vi "VelocityProfile.vi"(0 "t":dbl, 1 "a1":dbl=10.0, 3 "a3":dbl=15.0, 5 "s":dbl, 7 "intervalo":dbl=0.016, 9 "v_est":dbl, 11 "v_max":dbl=3.0, 12 "v3":dbl, 13 "s3":dbl) -> (4 "Velocity":dbl, 6 "VelocityProfileState Out":T1, 8 "Velocities":dbl[](array[numeric]), 10 "Time":dbl[](array[numeric]))   [LabVIEW 2018]
uses:
  Controle/VelocityProfileState.ctl
panel:
  in  "Amax":dbl=8.0
  in  "Reset":bool
  out "Velocity Profile":cluster{dbl[], dbl[]}(graph)
  in  "Tolerancia Vel":dbl=0.01
  in  "Tolerancia Pos":dbl=0.010000000000000004
  out "VelocityProfileState In":T1={"t0"=0.0, "t1"=0.0, "t2"=0.0, "t3"=0.0, "v0"=0.0, "v_max"=3.0, "v3"=0.0, "v2"=0.0, "v1"=0.0, "perfil"=enum."Triangular", "regiao"=0, "s0"=0.0, "s1"=0.0, "s2"=0.0, "v"=0.0, "t"=0.0, "a1"=10.0, "s3"=0.0, "Reset"=FALSE, "s"=0.0, "a3"=15.0, "Ré"=FALSE, "Impossível"=FALSE, "intervalo"=0.0}
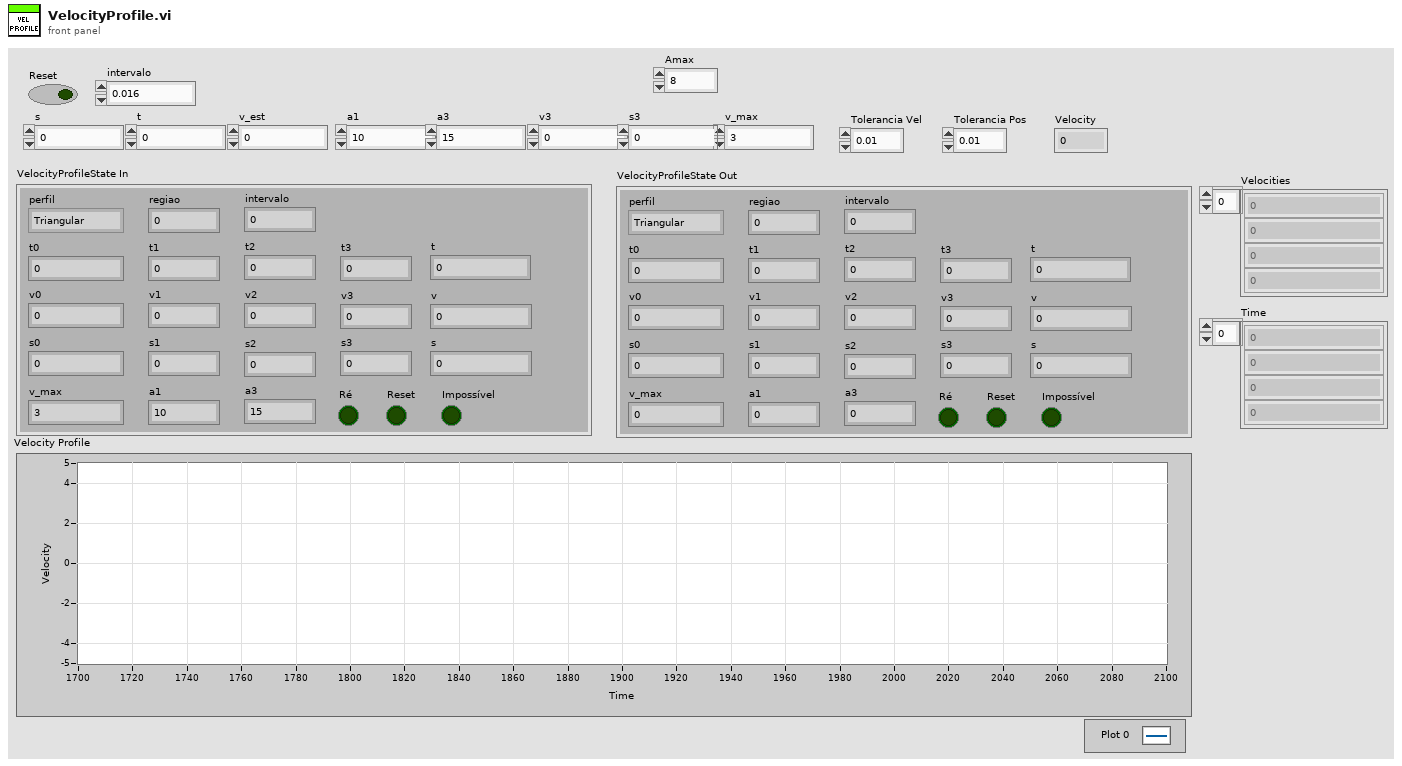
[diagram p1: front panel]
types:
  T1 = typedef "VelocityProfileState.ctl" = cluster{"t0":dbl, "t1":dbl, "t2":dbl, "t3":dbl, "v0":dbl, "v_max":dbl, "v3":dbl, "v2":dbl, "v1":dbl, "perfil":enum16{"Triangular", "Trapezoidal"}, "regiao":i32, "s0":dbl, "s1":dbl, "s2":dbl, "v":dbl, "t":dbl, "a1":dbl, "s3":dbl, "Reset":bool, "s":dbl, "a3":dbl, "Ré":bool, "Impossível":bool, "intervalo":dbl}
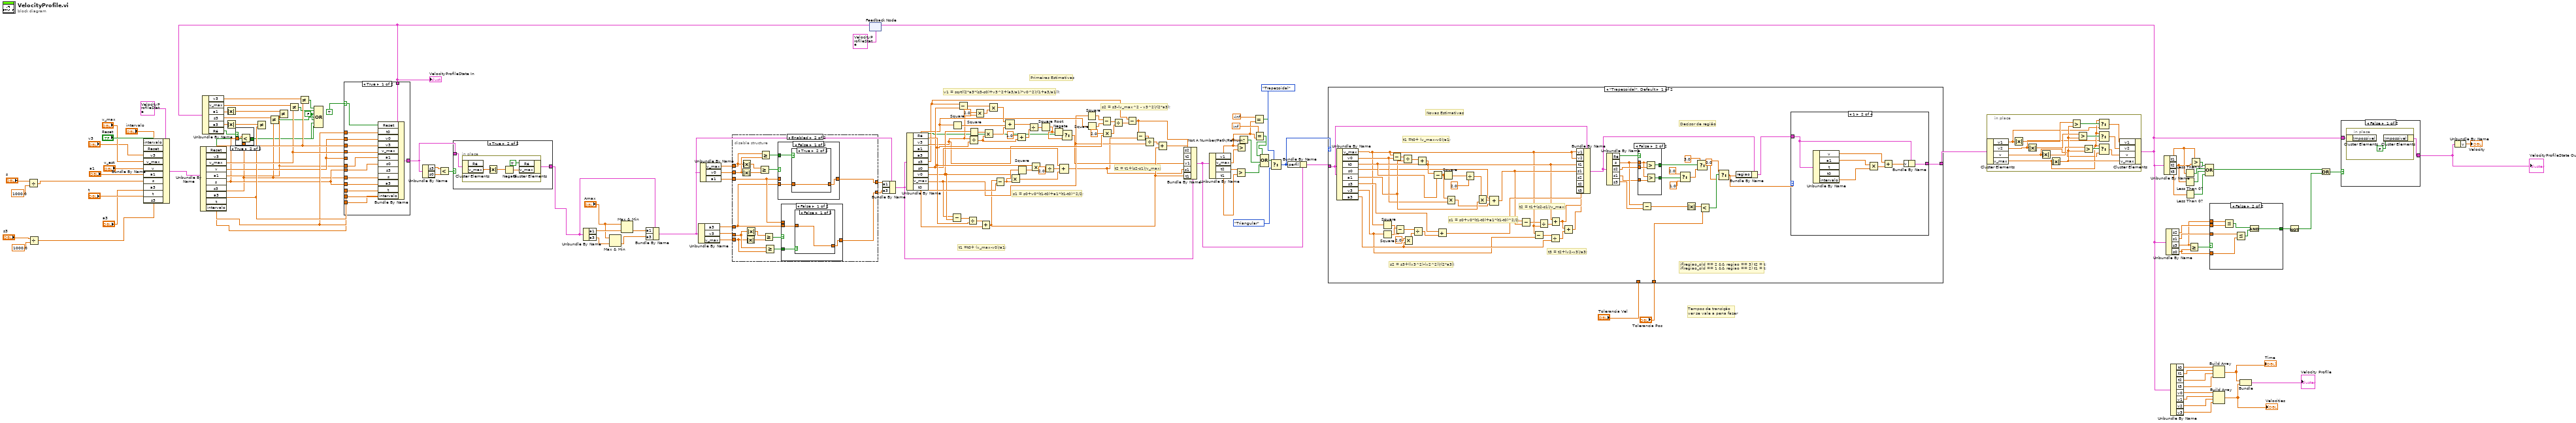
[diagram p0: block diagram]
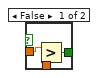
[diagram p2: hidden frame]
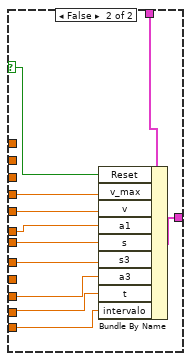
[diagram p3: hidden frame]
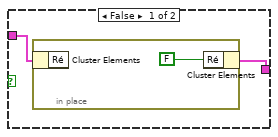
[diagram p4: hidden frame]
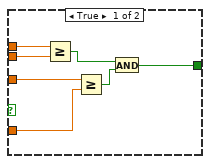
[diagram p5: hidden frame]
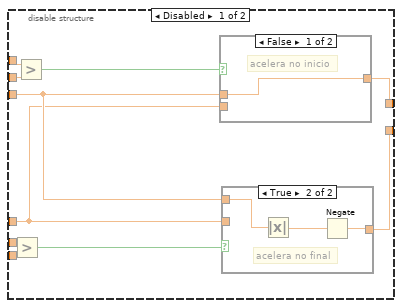
[diagram p6: hidden frame]
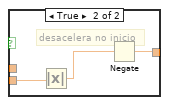
[diagram p8: hidden frame]
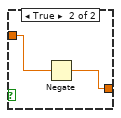
[diagram p9: hidden frame]
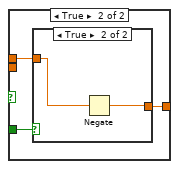
[diagram p10: hidden frame]
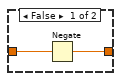
[diagram p12: hidden frame]
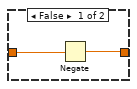
[diagram p14: hidden frame]
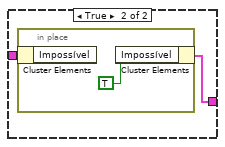
[diagram p15: hidden frame]
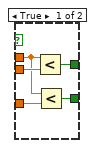
[diagram p16: hidden frame]
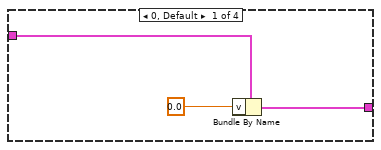
[diagram p17: hidden frame]
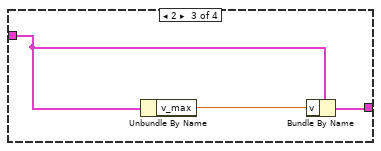
[diagram p18: hidden frame]
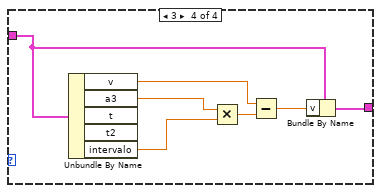
[diagram p19: hidden frame]
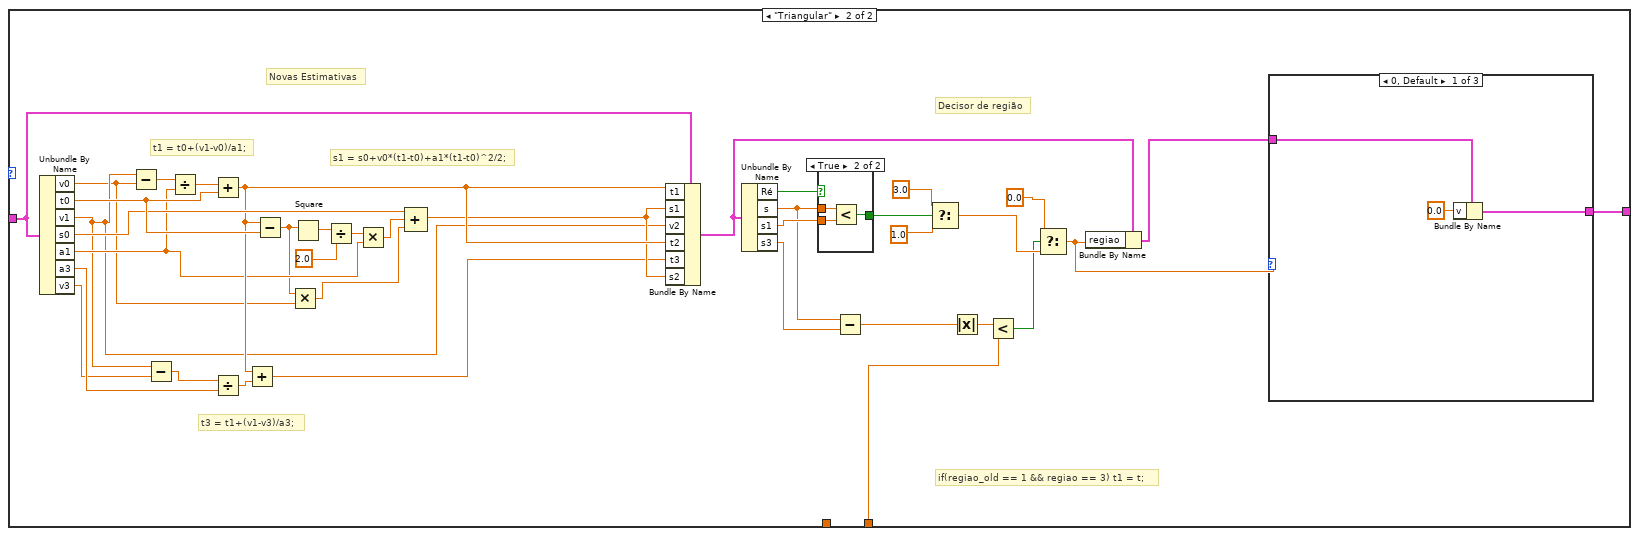
[diagram p20: hidden frame]
diagram:
  w37 = FALSE ("value")
  # "Tempos de transição\nver se vale a pena fazer"
  # "Primeiras Estimativas"
  # "t2 = t1+(s2-s1)/v_max;"
  # "s2 = s3-(v_max^2 - v3^2)/(2*a3);"
  # "s1 = s0+v0*(t1-t0)+a1*(t1-t0)^2/2;"
  # "t1 =t0+ (v_max-v0)/a1;"
  # "v1 = sqrt((2*a3*(s3-s0)+v3^2+(a3/a1)*v0^2)/(1+a3/a1));"
  n1 = Divide(x="s", y=1000.0) -> (x/y=w6:dbl)
  n2 = Divide(x="s3", y=1000.0) -> (x/y=w7:dbl)
  n3 = Bundle By Name(cluster=T1 {"t0"=0.0, "t1"=0.0, "t2"=0.0, "t3"=0.0, "v0"=0.0, "v_max"=0.0, "v3"=0.0, "v2"=0.0, "v1"=0.0, "perfil"=enum."Triangular", "regiao"=0, "s0"=0.0, "s1"=0.0, "s2"=0.0, "v"=0.0, "t"=0.0, "a1"=0.0, "s3"=0.0, "Reset"=FALSE, "s"=0.0, "a3"=0.0, "Ré"=FALSE, "Impossível"=FALSE, "intervalo"=0.0} ("VelocityProfileState In"), "intervalo"="intervalo", "Reset"="Reset", "v3"="v3", "v_max"="v_max", "v"="v_est", "a1"="a1", "s"=w6, "a3"="a3", "t"="t", "s3"=w7) -> (w43:T1)
  n4 = Unbundle By Name(w43) -> ("Reset"=w39:bool, "v3"=w135:dbl, "v_max"=w133:dbl, "v"=w63:dbl, "a1"=w62:dbl, "s"=w41:dbl, "s3"=w40:dbl, "a3"=w67:dbl, "t"=w64:dbl, "intervalo"=w31:dbl)
  n5 = feedback #1(T1 {"t0"=0.0, "t1"=0.0, "t2"=0.0, "t3"=0.0, "v0"=0.0, "v_max"=0.0, "v3"=0.0, "v2"=0.0, "v1"=0.0, "perfil"=enum."Triangular", "regiao"=0, "s0"=0.0, "s1"=0.0, "s2"=0.0, "v"=0.0, "t"=0.0, "a1"=0.0, "s3"=0.0, "Reset"=FALSE, "s"=0.0, "a3"=0.0, "Ré"=FALSE, "Impossível"=FALSE, "intervalo"=0.0} ("VelocityProfileState In")) -> (w19:T1)
  "VelocityProfileState In" <- w19
  n6 = Unbundle By Name(w19) -> ("v3"=w136:dbl, "v_max"=w134:dbl, "a1"=w46:dbl, "s3"=w132:dbl, "a3"=w45:dbl, "Ré"=w42:bool)
  n7 = Absolute Value(x=w46) -> (abs(x)=w47:dbl)
  n8 = Absolute Value(x=w45) -> (abs(x)=w44:dbl)
  n9 = case shown="True" w42 {
    tunnel: w41 -> [w158 w161]
    tunnel: w40 -> [w157 w160]
    tunnel: [w156 w159] -> w38
    frame False {
      n10 = Greater?(x=w158, y=w157) -> (0:w156:bool)
    }
    frame True {
      n11 = Less?(x=w161, y=w160) -> (x < y?=w159:bool)
    }
  }
  n12 = Not Equal?(x=w44, y=w67) -> ()  [unwired: 1 out]
  n13 = Not Equal?(x=w132, y=w40) -> (x != y?=w129:bool)
  n14 = Not Equal?(x=w47, y=w62) -> ()  [unwired: 1 out]
  n15 = Not Equal?(x=w134, y=w133) -> (x != y?=w130:bool)
  n16 = Not Equal?(x=w136, y=w135) -> (x != y?=w131:bool)
  n17 = Compound Arithmetic op=OR(w131, w130, w37, w129, w37, w38, w39) -> ()  [unwired: 1 out]
  n18 = case shown="True" TRUE {
    selector: TRUE -> [w169 w182]
    tunnel: w64 -> [w175 _]
    tunnel: w63 -> [w174 _]
    tunnel: w135 -> [w173 _]
    tunnel: w133 -> [w172 w186]
    tunnel: w63 -> [_ w185]
    tunnel: [w171 w184] -> w153
    tunnel: w19 -> [w170 w183]
    tunnel: w67 -> [w168 w181]
    tunnel: w64 -> [w167 w180]
    tunnel: w41 -> [w166 _]
    tunnel: w62 -> [w162 w179]
    tunnel: w41 -> [w165 w178]
    tunnel: w40 -> [w164 w177]
    tunnel: w31 -> [w163 w176]
    frame True {
      n19 = Bundle By Name(cluster=w170, "Reset"=w169, "t0"=w175, "v0"=w174, "v3"=w173, "v_max"=w172, "a1"=w162, "s0"=w165, "s3"=w164, "s"=w166, "a3"=w168, "t"=w167, "intervalo"=w163) -> (w171:T1)
    }
    frame False {
      n20 = Bundle By Name(cluster=w183, "Reset"=w182, "v_max"=w186, "v"=w185, "a1"=w179, "s"=w178, "s3"=w177, "a3"=w181, "t"=w180, "intervalo"=w176) -> (w184:T1)
    }
  }
  n21 = Unbundle By Name(w153) -> ("s3"=w155:dbl, "s0"=w154:dbl)
  n22 = Less?(x=w155, y=w154) -> (x < y?=w66:bool)
  n23 = case shown="True" w66 {
    tunnel: w153 -> [w188 w191]
    tunnel: [w187 w190] -> w15
    frame False {
      n24 = in-place {
        n25 = in-place-cluster #2(w188) -> ()  [unwired: 1 out]
        n26 = in-place-cluster #2("Ré"=FALSE) -> (w187:T1)
      }
    }
    frame True {
      n27 = in-place {
        n28 = in-place-cluster #3(w191) -> ("v_max"=w195:dbl)  [unwired: 1 out]
        n29 = Absolute Value(x=w195) -> (abs(x)=w194:dbl)
        n30 = Negate(x=w194) -> (-x=w193:dbl)
        n31 = in-place-cluster #3("Ré"=TRUE, "v_max"=w193) -> (w190:T1)
      }
    }
  }
  n32 = Unbundle By Name(w15) -> ("a1"=w14:dbl, "a3"=w11:dbl)
  n33 = Max & Min(x="Amax", y=w11) -> (min(x,y)=w10:dbl)  [unwired: 1 out]
  n34 = Max & Min(x="Amax", y=w14) -> (min(x,y)=w13:dbl)  [unwired: 1 out]
  n35 = Bundle By Name(cluster=w15, "a1"=w13, "a3"=w10) -> (w16:T1)
  n36 = Unbundle By Name(w16) -> ("a3"=w68:dbl, "v3"=w113:dbl, "v_max"=w114:dbl)
  n37 = Unbundle By Name(w16) -> ("v_max"=w152:dbl, "v0"=w151:dbl, "a1"=w69:dbl)
  n38 = disable-structure shown="Enabled" {
    disable-tunnel: w152 -> [w205 w225]
    disable-tunnel: w151 -> [w204 w224]
    disable-tunnel: w114 -> [w203 w216]
    disable-tunnel: w113 -> [w202 w217]
    disable-tunnel: [w200 w223] -> w71
    disable-tunnel: [w198 w218] -> w70
    disable-tunnel: w69 -> [w197 w215]
    disable-tunnel: w68 -> [w196 w214]
    frame Disabled {
      n39 = Greater?(x=w202, y=w203) -> (0:w199:bool)
      n40 = Greater?(x=w205, y=w204) -> (0:w201:bool)
      n41 = case shown="False" w201 {
        tunnel: [w210 w212] -> w200
        tunnel: w197 -> [w210 _]
        tunnel: w196 -> [_ w213]
        frame False {
          # "acelera no inicio"
        }
        frame True {
          # "desacelera no inicio"
          n42 = Absolute Value(x=w213) -> (abs(x)=w211:dbl)
          n43 = Negate(x=w211) -> (-x=w212:dbl)
        }
      }
      n44 = case shown="True" w199 {
        tunnel: [w206 w209] -> w198
        tunnel: w197 -> [_ w207]
        tunnel: w196 -> [w206 _]
        frame False {
          # "desacelera no final"
        }
        frame True {
          # "acelera no final"
          n45 = Absolute Value(x=w207) -> (abs(x)=w208:dbl)
          n46 = Negate(x=w208) -> (-x=w209:dbl)
        }
      }
    }
    frame Enabled {
      n47 = Absolute Value(x=w224) -> (abs(x)=w228:dbl)
      n48 = Absolute Value(x=w225) -> (abs(x)=w229:dbl)
      n49 = Absolute Value(x=w216) -> (abs(x)=w220:dbl)
      n50 = Absolute Value(x=w217) -> (abs(x)=w219:dbl)
      n51 = Greater Or Equal?(x=w229, y=w228) -> (x >= y?=w227:bool)
      n52 = Greater Or Equal?(x=w225, y=w224) -> (x >= y?=w226:bool)
      n53 = Greater Or Equal?(x=w219, y=w220) -> (x >= y?=w221:bool)
      n54 = Greater Or Equal?(x=w217, y=w216) -> (x >= y?=w222:bool)
      n55 = case shown="False" w227 {
        tunnel: w215 -> [_ w248]
        tunnel: w226 -> [w244 w250]
        tunnel: [w243 w249] -> w223
        tunnel: w214 -> [w242 _]
        frame False {
          n56 = case shown="True" w244 {
            tunnel: [w245 w247] -> w243
            tunnel: w242 -> [w246 w247]
            frame False {
              n57 = Negate(x=w246) -> (-x=w245:dbl)
            }
            frame True {
            }
          }
        }
        frame True {
          n58 = case shown="True" w250 {
            tunnel: [w251 w253] -> w249
            tunnel: w248 -> [w252 w253]
            frame False {
              n59 = Negate(x=w252) -> (-x=w251:dbl)
            }
            frame True {
            }
          }
        }
      }
      n60 = case shown="False" w221 {
        tunnel: w222 -> [w232 w238]
        tunnel: [w231 w237] -> w218
        tunnel: w215 -> [_ w236]
        tunnel: w214 -> [w230 _]
        frame False {
          n61 = case shown="False" w232 {
            tunnel: [w233 w234] -> w231
            tunnel: w230 -> [w233 w235]
            frame False {
            }
            frame True {
              n62 = Negate(x=w235) -> (-x=w234:dbl)
            }
          }
        }
        frame True {
          n63 = case shown="True" w238 {
            tunnel: [w239 w241] -> w237
            tunnel: w236 -> [w239 w240]
            frame False {
            }
            frame True {
              n64 = Negate(x=w240) -> (-x=w241:dbl)
            }
          }
        }
      }
    }
  }
  n65 = Bundle By Name(cluster=w16, "a1"=w71, "a3"=w70) -> (w72:T1)
  n66 = Unbundle By Name(w72) -> ("Ré"=w65:bool, "v3"=w87:dbl, "a1"=w105:dbl, "a3"=w84:dbl, "s3"=w81:dbl, "s0"=w104:dbl, "v0"=w103:dbl, "v_max"=w79:dbl, "t0"=w112:dbl)
  n67 = Subtract(x=w79, y=w103) -> (x-y=w150:dbl)
  n68 = Square(x=w87) -> (x^2=w100:dbl)
  n69 = Subtract(x=w81, y=w104) -> (x-y=w99:dbl)
  n70 = Divide(x=w150, y=w105) -> (x/y=w149:dbl)
  n71 = Divide(x=w84, y=w105) -> (x/y=w93:dbl)
  n72 = Square(x=w103) -> (x^2=w102:dbl)
  n73 = Multiply(x=2.0, y=w84) -> (x*y=w98:dbl)
  n74 = Add(x=w149, y=w112) -> (x+y=w77:dbl)
  n75 = Multiply(x=w102, y=w93) -> (x*y=w101:dbl)
  n76 = Multiply(x=w99, y=w98) -> (x*y=w96:dbl)
  n77 = Subtract(x=w77, y=w112) -> (x-y=w111:dbl)
  n78 = Compound Arithmetic op=ADD(w96, w100, w101) -> (w95:dbl)
  n79 = Multiply(x=w103, y=w111) -> (x*y=w106:dbl)
  n80 = Add(x=1.0, y=w93) -> (x+y=w94:dbl)
  n81 = Square(x=w111) -> (x^2=w110:dbl)
  n82 = Divide(x=w95, y=w94) -> (x/y=w91:dbl)
  n83 = Multiply(x=w105, y=w110) -> (x*y=w109:dbl)
  n84 = Square Root(x=w91) -> (sqrt(x)=w90:dbl)
  n85 = Divide(x=w109, y=2.0) -> (x/y=w107:dbl)
  n86 = Negate(x=w90) -> (-x=w117:dbl)
  n87 = Compound Arithmetic op=ADD(w104, w107, w106) -> (w73:dbl)
  n88 = Select(t=w117, s=w65, f=w90) -> (s? t:f=w74:dbl)
  n89 = Square(x=w79) -> (x^2=w89:dbl)
  n90 = Square(x=w87) -> (x^2=w88:dbl)
  n91 = Subtract(x=w89, y=w88) -> (x-y=w86:dbl)
  n92 = Multiply(x=2.0, y=w84) -> (x*y=w85:dbl)
  n93 = Divide(x=w86, y=w85) -> (x/y=w82:dbl)
  n94 = Subtract(x=w81, y=w82) -> (x-y=w76:dbl)
  n95 = Subtract(x=w76, y=w73) -> (x-y=w80:dbl)
  n96 = Divide(x=w80, y=w79) -> (x/y=w78:dbl)
  n97 = Add(x=w78, y=w77) -> (x+y=w75:dbl)
  n98 = Bundle By Name(cluster=w72, "s2"=w76, "t2"=w75, "v1"=w74, "s1"=w73, "t1"=w77) -> (w141:T1)
  n99 = Unbundle By Name(w141) -> ("v1"=w3:dbl, "v_max"=w148:dbl, "t2"=w147:dbl, "t1"=w146:dbl)
  n100 = Greater?(x=w147, y=w146) -> (0:w36:bool)
  n101 = Greater?(x=w3, y=w148) -> ()  [unwired: 1 out]
  n102 = Not A Number/Path/Refnum?(number/path/refnum=w3) -> (NaN/Path/Refnum?=w115:bool)
  n103 = Equal?(x=-inf, y=w3) -> (x = y?=w1:bool)
  n104 = Equal?(x=inf, y=w3) -> (x = y?=w35:bool)
  n105 = Compound Arithmetic op=OR(w1, w35, w115, w36) -> (w116:bool)
  n106 = Select(t=enum16{"Triangular", "Trapezoidal"}."Trapezoidal" ("perfil"), s=w116, f=enum16{"Triangular", "Trapezoidal"}."Triangular" ("perfil")) -> (s? t:f=w143:enum16{"Triangular", "Trapezoidal"})
  n107 = Bundle By Name(cluster=w141, "perfil"=w143) -> (w142:T1)
  n108 = case shown="\"Trapezoidal\", Default" w143 {
    tunnel: w142 -> [w306 w366]
    tunnel: [w294 w353] -> w138
    tunnel: "Tolerancia Pos" -> [w277 w351]
    tunnel: "Tolerancia Vel" -> [_ _]
    frame "Trapezoidal", Default {
      # "t3 = t2+(v2-v3)/a3;"
      # "t2 = t1+(s2-s1)/v_max;"
      # "s2 = s3+((v3^2)-(v2^2))/(2*a3);"
      # "s1 = s0+v0*(t1-t0)+a1*(t1-t0)^2/2;"
      # "t1 =t0+ (v_max-v0)/a1;"
      # "if(regiao_old == 2 && regiao == 3) t2 = t;\nif(regiao_old == 1 && regiao == 2) t1 = t;"
      # "Decisor de região"
      # "Novas Estimativas"
      n109 = Unbundle By Name(w306) -> ("v_max"=w259:dbl, "v0"=w271:dbl, "t0"=w281:dbl, "s0"=w270:dbl, "a1"=w280:dbl, "s3"=w261:dbl, "v3"=w257:dbl, "a3"=w264:dbl)
      n110 = Square(x=w259) -> (x^2=w267:dbl)
      n111 = Square(x=w257) -> (x^2=w268:dbl)
      n112 = Subtract(x=w259, y=w271) -> (x-y=w293:dbl)
      n113 = Subtract(x=w268, y=w267) -> (x-y=w266:dbl)
      n114 = Divide(x=w293, y=w280) -> (x/y=w292:dbl)
      n115 = Multiply(x=2.0, y=w264) -> (x*y=w265:dbl)
      n116 = Divide(x=w266, y=w265) -> (x/y=w262:dbl)
      n117 = Add(x=w292, y=w281) -> (x+y=w284:dbl)
      n118 = Subtract(x=w284, y=w281) -> (x-y=w272:dbl)
      n119 = Add(x=w261, y=w262) -> (x+y=w287:dbl)
      n120 = Square(x=w272) -> (x^2=w291:dbl)
      n121 = Multiply(x=w272, y=w271) -> (x*y=w269:dbl)
      n122 = Divide(x=w291, y=2.0) -> (x/y=w289:dbl)
      n123 = Multiply(x=w289, y=w280) -> (x*y=w288:dbl)
      n124 = Compound Arithmetic op=ADD(w270, w288, w269) -> (w286:dbl)
      n125 = Subtract(x=w287, y=w286) -> (x-y=w260:dbl)
      n126 = Subtract(x=w259, y=w257) -> (x-y=w258:dbl)
      n127 = Divide(x=w260, y=w259) -> (x/y=w285:dbl)
      n128 = Divide(x=w258, y=w264) -> (x/y=w282:dbl)
      n129 = Add(x=w284, y=w285) -> (x+y=w283:dbl)
      n130 = Add(x=w283, y=w282) -> (x+y=w279:dbl)
      n131 = Bundle By Name(cluster=w306, "v1"=w259, "v2"=w259, "t1"=w284, "s1"=w286, "s2"=w287, "t2"=w283, "t3"=w279) -> (w297:T1)
      n132 = Unbundle By Name(w297) -> ("Ré"=w256:bool, "s"=w302:dbl, "s2"=w305:dbl, "s1"=w255:dbl, "s3"=w276:dbl)
      n133 = case shown="False" w256 {
        tunnel: w305 -> [w311 w316]
        tunnel: [w310 w315] -> w304
        tunnel: w302 -> [w309 w314]
        tunnel: w255 -> [w308 w313]
        tunnel: [w307 w312] -> w254
        frame True {
          n134 = Less?(x=w309, y=w311) -> (x < y?=w310:bool)
          n135 = Less?(x=w309, y=w308) -> (x < y?=w307:bool)
        }
        frame False {
          n136 = Greater?(x=w314, y=w316) -> (0:w315:bool)
          n137 = Greater?(x=w314, y=w313) -> (0:w312:bool)
        }
      }
      n138 = Subtract(x=w302, y=w276) -> (x-y=w301:dbl)
      n139 = Select(t=2.0, s=w254, f=1.0) -> (s? t:f=w273:dbl)
      n140 = Absolute Value(x=w301) -> (abs(x)=w300:dbl)
      n141 = Select(t=3.0, s=w304, f=w273) -> (s? t:f=w278:dbl)
      n142 = Less?(x=w300, y=w277) -> (x < y?=w299:bool)
      n143 = Select(t=0.0, s=w299, f=w278) -> (s? t:f=w296:dbl)
      n144 = Bundle By Name(cluster=w297, "regiao"=w296) -> (w295:T1)
      n145 = case shown="1" w296 {
        tunnel: w295 -> [w319 w326 w328 w336]
        tunnel: [w317 w325 w329 w335] -> w294
        frame 0, Default {
          n146 = Bundle By Name(cluster=w319, "v"=0.0) -> (w317:T1)
        }
        frame 1 {
          n147 = Unbundle By Name(w326) -> ("v"=w322:dbl, "a1"=w324:dbl, "intervalo"=w320:dbl)  [unwired: 2 out]
          n148 = Multiply(x=w324, y=w320) -> (x*y=w323:dbl)
          n149 = Add(x=w322, y=w323) -> (x+y=w321:dbl)
          n150 = Bundle By Name(cluster=w326, "v"=w321) -> (w325:T1)
        }
        frame 2 {
          n151 = Unbundle By Name(w328) -> ("v_max"=w327:dbl)
          n152 = Bundle By Name(cluster=w328, "v"=w327) -> (w329:T1)
        }
        frame 3 {
          n153 = Unbundle By Name(w336) -> ("v"=w332:dbl, "a3"=w334:dbl, "intervalo"=w330:dbl)  [unwired: 2 out]
          n154 = Multiply(x=w334, y=w330) -> (x*y=w333:dbl)
          n155 = Subtract(x=w332, y=w333) -> (x-y=w331:dbl)
          n156 = Bundle By Name(cluster=w336, "v"=w331) -> (w335:T1)
        }
      }
    }
    frame "Triangular" {
      # "if(regiao_old == 1 && regiao == 3) t1 = t;"
      # "Decisor de região"
      # "Novas Estimativas"
      # "t3 = t1+(v1-v3)/a3;"
      # "s1 = s0+v0*(t1-t0)+a1*(t1-t0)^2/2;"
      # "t1 = t0+(v1-v0)/a1;"
      n157 = Unbundle By Name(w366) -> ("v0"=w339:dbl, "t0"=w372:dbl, "v1"=w343:dbl, "s0"=w369:dbl, "a1"=w346:dbl, "a3"=w345:dbl, "v3"=w342:dbl)
      n158 = Subtract(x=w343, y=w339) -> (x-y=w374:dbl)
      n159 = Subtract(x=w343, y=w342) -> (x-y=w344:dbl)
      n160 = Divide(x=w374, y=w346) -> (x/y=w373:dbl)
      n161 = Add(x=w373, y=w372) -> (x+y=w367:dbl)
      n162 = Divide(x=w344, y=w345) -> (x/y=w368:dbl)
      n163 = Add(x=w367, y=w368) -> (x+y=w341:dbl)
      n164 = Subtract(x=w367, y=w372) -> (x-y=w340:dbl)
      n165 = Multiply(x=w340, y=w339) -> (x*y=w338:dbl)
      n166 = Square(x=w340) -> (x^2=w371:dbl)
      n167 = Divide(x=w371, y=2.0) -> (x/y=w348:dbl)
      n168 = Multiply(x=w348, y=w346) -> (x*y=w347:dbl)
      n169 = Compound Arithmetic op=ADD(w369, w347, w338) -> (w352:dbl)
      n170 = Bundle By Name(cluster=w366, "t1"=w367, "s1"=w352, "v2"=w343, "t2"=w367, "t3"=w341, "s2"=w352) -> (w356:T1)
      n171 = Unbundle By Name(w356) -> ("Ré"=w337:bool, "s"=w362:dbl, "s1"=w365:dbl, "s3"=w361:dbl)
      n172 = case shown="True" w337 {
        tunnel: w365 -> [w377 w378]
        tunnel: [w376 w380] -> w364
        tunnel: w362 -> [w375 w379]
        frame False {
          n173 = Greater?(x=w375, y=w377) -> (0:w376:bool)
        }
        frame True {
          n174 = Less?(x=w379, y=w378) -> (x < y?=w380:bool)
        }
      }
      n175 = Subtract(x=w362, y=w361) -> (x-y=w360:dbl)
      n176 = Select(t=3.0, s=w364, f=1.0) -> (s? t:f=w358:dbl)
      n177 = Absolute Value(x=w360) -> (abs(x)=w359:dbl)
      n178 = Less?(x=w359, y=w351) -> (x < y?=w357:bool)
      n179 = Select(t=0.0, s=w357, f=w358) -> (s? t:f=w355:dbl)
      n180 = Bundle By Name(cluster=w356, "regiao"=w355) -> (w354:T1)
      n181 = case shown="0, Default" w355 {
        tunnel: w354 -> [w383 w390 w397]
        tunnel: [w381 w389 w396] -> w353
        frame 0, Default {
          n182 = Bundle By Name(cluster=w383, "v"=0.0) -> (w381:T1)
        }
        frame 1 {
          n183 = Unbundle By Name(w390) -> ("v"=w386:dbl, "a1"=w388:dbl, "intervalo"=w384:dbl)  [unwired: 2 out]
          n184 = Multiply(x=w388, y=w384) -> (x*y=w387:dbl)
          n185 = Add(x=w386, y=w387) -> (x+y=w385:dbl)
          n186 = Bundle By Name(cluster=w390, "v"=w385) -> (w389:T1)
        }
        frame 3 {
          n187 = Unbundle By Name(w397) -> ("v"=w393:dbl, "a3"=w395:dbl, "intervalo"=w391:dbl)  [unwired: 2 out]
          n188 = Multiply(x=w395, y=w391) -> (x*y=w394:dbl)
          n189 = Subtract(x=w393, y=w394) -> (x-y=w392:dbl)
          n190 = Bundle By Name(cluster=w397, "v"=w392) -> (w396:T1)
        }
      }
    }
  }
  n191 = in-place {
    n192 = in-place-cluster #4(w138) -> ("v1"=w400:dbl, "v2"=w399:dbl, "v"=w398:dbl, "v_max"=w401:dbl)
    n193 = Absolute Value(x=w400) -> (abs(x)=w406:dbl)
    n194 = Absolute Value(x=w399) -> (abs(x)=w405:dbl)
    n195 = Absolute Value(x=w398) -> (abs(x)=w404:dbl)
    n196 = Absolute Value(x=w401) -> (abs(x)=w403:dbl)
    n197 = Greater?(x=w406, y=w403) -> (0:w411:bool)
    n198 = Greater?(x=w405, y=w403) -> (0:w410:bool)
    n199 = Greater?(x=w404, y=w403) -> (0:w402:bool)
    n200 = Select(t=w401, s=w411, f=w400) -> (s? t:f=w409:dbl)
    n201 = Select(t=w401, s=w410, f=w399) -> (s? t:f=w408:dbl)
    n202 = Select(t=w401, s=w402, f=w398) -> (s? t:f=w407:dbl)
    n203 = in-place-cluster #4("v1"=w409, "v2"=w408, "v"=w407, "v_max"=w403) -> (w30:T1)
  }
  n204 = feedback-in #1(w30) -> ()
  n205 = Unbundle By Name(w30) -> ("t1"=w58:dbl, "t2"=w18:dbl, "t3"=w55:dbl)
  n206 = Unbundle By Name(w30) -> ("s2"=w26:dbl, "s1"=w28:dbl, "s3"=w25:dbl, "s0"=w27:dbl)
  n207 = Unbundle By Name(w30) -> ("t0"=w127:dbl, "t1"=w126:dbl, "t2"=w125:dbl, "t3"=w124:dbl, "v0"=w123:dbl, "v1"=w122:dbl, "v2"=w121:dbl, "v3"=w120:dbl)
  n208 = Less Than 0?(x=w58) -> (x < 0?=w57:bool)
  n209 = Less Than 0?(x=w18) -> (x < 0?=w56:bool)
  n210 = Less Than 0?(x=w55) -> (x < 0?=w54:bool)
  n211 = Greater Or Equal?(x=w25, y=w27) -> (x >= y?=w29:bool)
  n212 = Greater?(x=w58, y=w18) -> (0:w17:bool)
  n213 = Compound Arithmetic op=OR(w17, w57, w56, w54) -> (w23:bool)
  n214 = case shown="False" w29 {
    tunnel: w28 -> [w417 w424]
    tunnel: w27 -> [w418 w425]
    tunnel: w26 -> [w416 w423]
    tunnel: w25 -> [w415 w422]
    tunnel: [w412 w419] -> w22
    frame True {
      n215 = Greater Or Equal?(x=w415, y=w416) -> (x >= y?=w413:bool)
      n216 = Greater Or Equal?(x=w417, y=w418) -> (x >= y?=w414:bool)
      n217 = And(x=w413, y=w414) -> (x .and. y?=w412:bool)
    }
    frame False {
      n218 = Less Or Equal?(x=w422, y=w423) -> (x <= y?=w420:bool)
      n219 = Less Or Equal?(x=w424, y=w425) -> (x <= y?=w421:bool)
      n220 = And(x=w420, y=w421) -> (x .and. y?=w419:bool)
    }
  }
  n221 = Build Array(w127, w126, w125, w124) -> (w119:dbl[])
  "Time" <- w119
  n222 = Build Array(w123, w122, w121, w120) -> (w118:dbl[])
  "Velocities" <- w118
  n223 = Bundle(w119, w118) -> (→"Velocity Profile":cluster{dbl[], dbl[]})  [unwired: 1 in]
  n224 = Not(x=w22) -> (.not. x?=w21:bool)
  n225 = Or(x=w23, y=w21) -> (x .or. y?=w24:bool)
  n226 = case shown="False" w24 {
    tunnel: w30 -> [w427 w430]
    tunnel: [w426 w429] -> w53
    frame False {
      n227 = in-place {
        n228 = in-place-cluster #5(w427) -> ()  [unwired: 1 out]
        n229 = in-place-cluster #5("Impossível"=FALSE) -> (w426:T1)
      }
    }
    frame True {
      n230 = in-place {
        n231 = in-place-cluster #6(w430) -> ()  [unwired: 1 out]
        n232 = in-place-cluster #6("Impossível"=TRUE) -> (w429:T1)
      }
    }
  }
  "VelocityProfileState Out" <- w53
  n233 = Unbundle By Name(w53) -> ("v"=→"Velocity":dbl)
